vi "dataBuffer HRT.vi"(4 "all data in":T1[](array[typedef]), 6 "command":T2=enum."read recent", 8 "error in (no error)":errorcluster, 10 "max array size":u16=5000 min=1, 11 "averaged data":T1) -> (0 "error out":errorcluster, 1 "all data out":T1[](array[typedef]), 2 "scans":i32, 3 "recent data":T1)   [LabVIEW 2015]
uses:
  data cluster.ctl
  Sensor buffer command.ctl
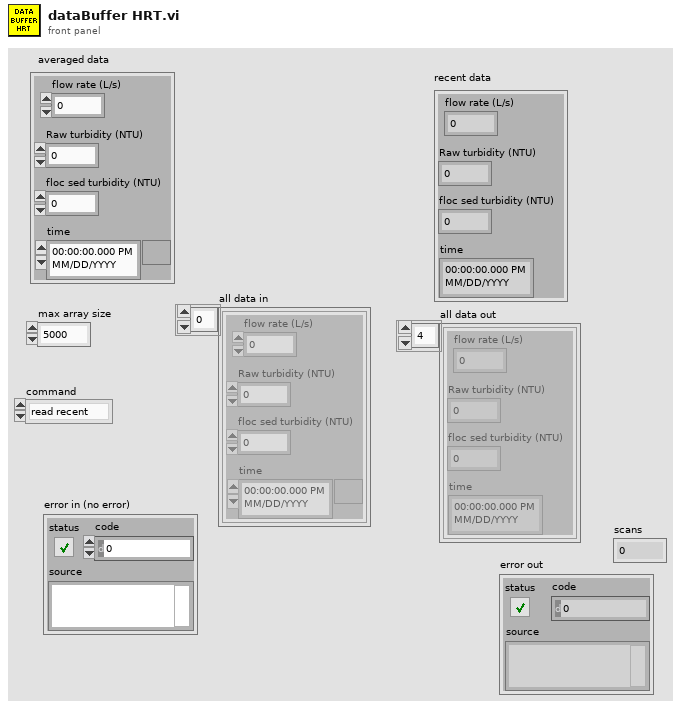
[diagram p1: front panel]
types:
  T1 = typedef "data cluster.ctl" = cluster{"floc sed turbidity (NTU)":dbl, "Raw turbidity (NTU)":dbl, "flow rate (L/s)":dbl, "time":timestamp}
  T2 = typedef "Sensor buffer command.ctl" = enum16{"set buffer size", "write", "refill buffer", "read recent", "read all", "clear"}
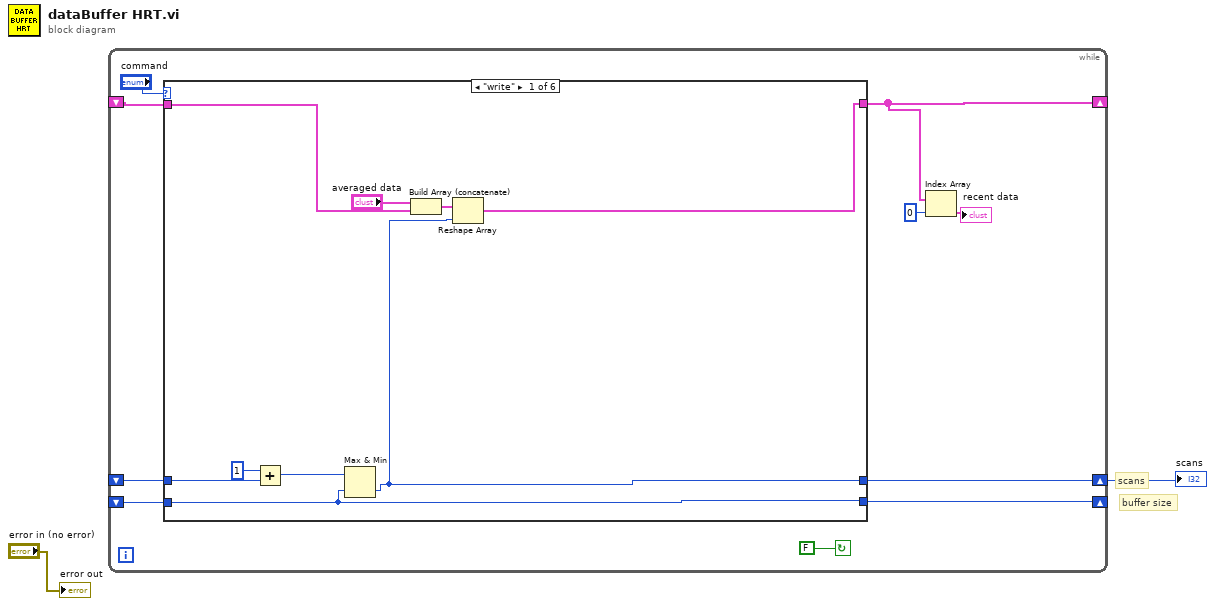
[diagram p0: block diagram]
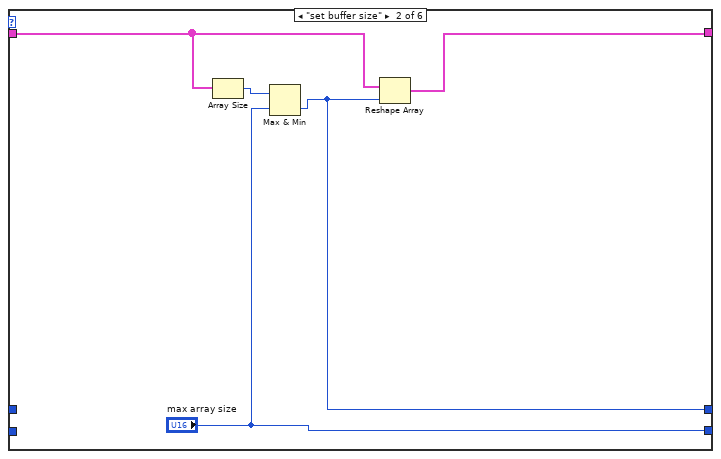
[diagram p2: hidden frame]
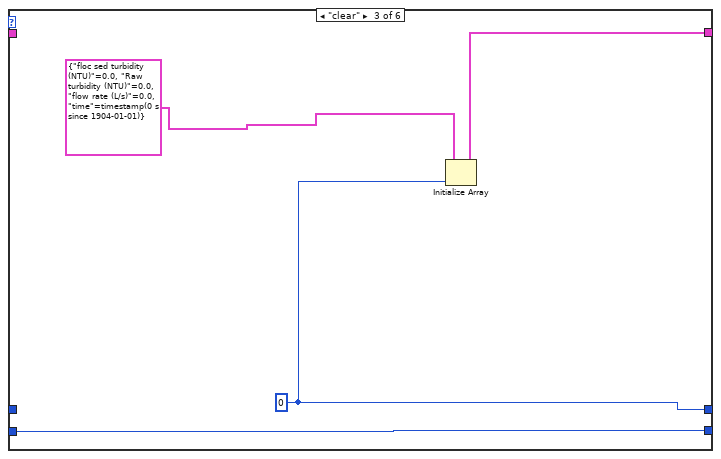
[diagram p3: hidden frame]
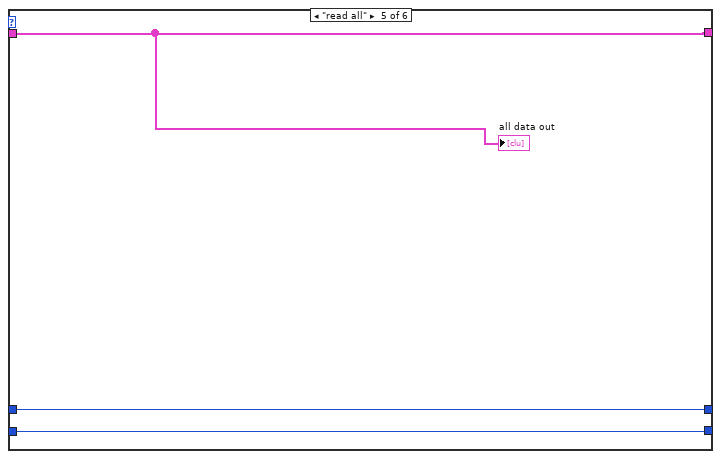
[diagram p5: hidden frame]
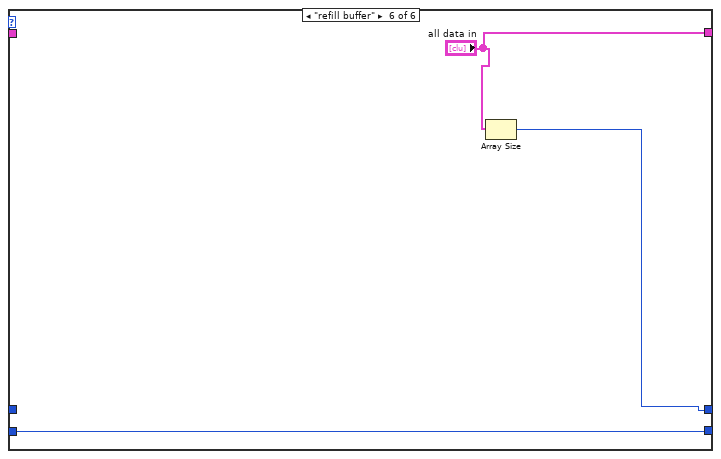
[diagram p6: hidden frame]
diagram:
  # "buffer size"
  # "scans"
  n1 = while {
    shift-right: [w3] -> _
    shift-left: _ -> [w11]
    shift-right: [w10] -> _
    shift-left: _ -> [w9]
    shift-right: [w6] -> w1
    shift-left: _ -> [w7]
    stop <- FALSE continue-if-true
    n2 = case shown="\"write\"" "command" {
      tunnel: [w18 w26 w30 w33 w34 "all data in"] -> w3
      tunnel: w11 -> [w20 w25 _ w33 w34 _]
      tunnel: [w16 "max array size" w29 w32 w36 w39] -> w10
      tunnel: w9 -> [w16 _ w29 w32 w36 w39]
      tunnel: w7 -> [w19 _ _ w31 w35 _]
      tunnel: [w13 w22 w27 w31 w35 w37] -> w6
      frame "write" {
        n3 = Add(x=1, y=w19) -> (x+y=w15:i32)
        n4 = Max & Min(x=w15, y=w16) -> (min(x,y)=w13:i32)  [unwired: 1 out]
        n5 = Build Array (concatenate)("averaged data", w20) -> (w17:T1[])
        n6 = Reshape Array(w17, w13) -> (w18:T1[])
      }
      frame "set buffer size" {
        n7 = Array Size(array=w25) -> (size(s)=w24:i32)
        n8 = Max & Min(x=w24, y="max array size") -> (min(x,y)=w22:i32)  [unwired: 1 out]
        n9 = Reshape Array(w25, w22) -> (w26:T1[])
      }
      frame "clear" {
        w27 = 0
        n10 = Initialize Array(T1 {"floc sed turbidity (NTU)"=0.0, "Raw turbidity (NTU)"=0.0, "flow rate (L/s)"=0.0, "time"=timestamp(0 s since 1904-01-01)} ("Calibrated data"), w27) -> (w30:T1[])
      }
      frame "read recent" {
      }
      frame "read all" {
        "all data out" <- w34
      }
      frame "refill buffer" {
        n11 = Array Size(array="all data in") -> (size(s)=w37:i32)
      }
    }
    n12 = Index Array(array=w3, index=0) -> (element=→"recent data":T1)
  }
  "scans" <- w1
  "error out" <- "error in (no error)"
